vi "Periodic Tasks.vi"(8 "error in":errorcluster) -> ()   [LabVIEW 2016]
doc: "This VI runs in parallel to other tasks. It can contain as many user-defined periodic loops as you need. These can carry out PID or other sorts of timed response."
uses:
  <vilib>/Rock Robotics/WPI/DriverStation/WPI_DriverStationRobotMode2.ctl
  <vilib>/Rock Robotics/WPI/Utilities/WPI_GetSetVariantRefNum.vi
  <vilib>/Rock Robotics/Network Tables/NT Write Number.vi
  <vilib>/Instr/_visa.llb/VISA Configure Serial Port (Instr).vi
  Systems/Global 1.vi
  Global 2.vi
panel:
  in  "Gyro Reset":bool
  out "Angle":dbl
  in  "Reset Drive":bool
  out "Waveform Chart":dbl(graph)
  out "PSI":dbl=101.0986199
  out "Shoot 0":dbl format="%#_13g"
  out "Shoot 1":dbl format="%#_13g"
  out "read buffer":string="B:2,X:203.00"
  in  "Search_Params":string[](array[string])=["B", "X", "Y", "W1", "H1", "W2", "H2"]
  out "Last Complete Message":string="B:2,X:203.00,Y:125.00,W1:11,H1:27,W2:8,H2:25"
  out "length":i32=44
  in  "off set":dbl format="%#_13g"
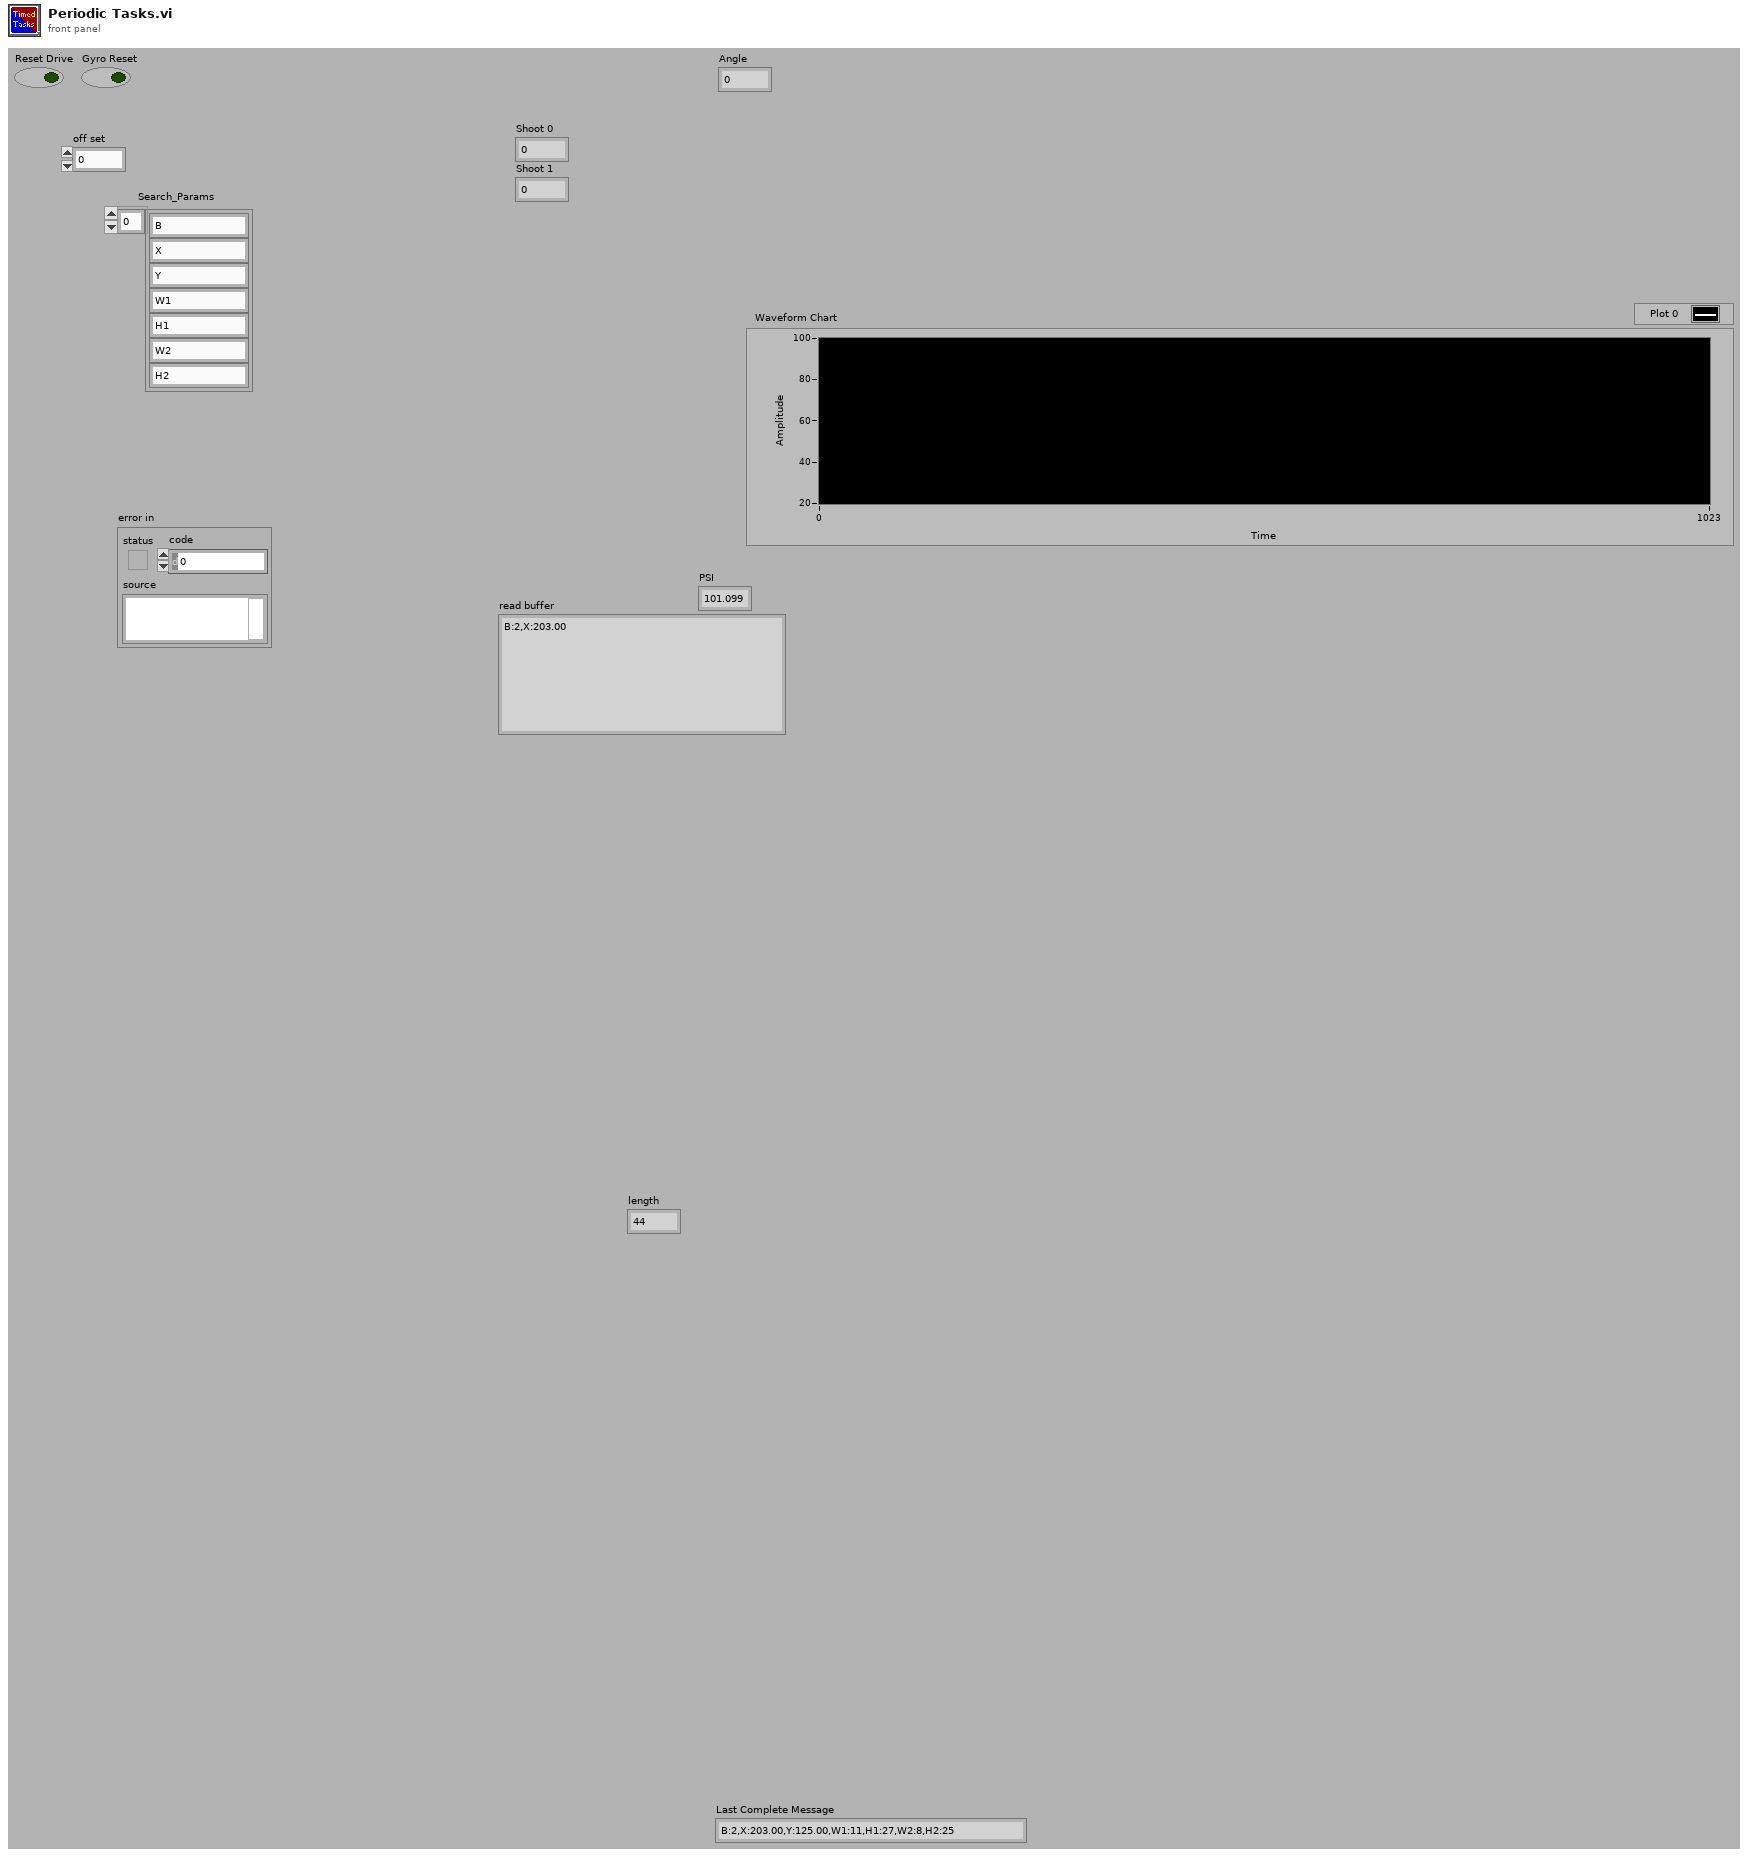
[diagram p1: front panel]
types:
  T1 = typedef "WPI_JoystickDevRef.ctl" = cluster{"Device":T2}
  T2 = typedef "WPI_JoystickDeviceEnum.ctl" = enum16{"USB 0", "USB 1", "USB 2", "USB 3", "USB 4", "USB 5"}
  T3 = typedef "WPI_MotorControlDeviceRef.ctl" = cluster{"DeviceStatus":errorcluster, "Type":T4, "PWM":cluster{"PWM Channel":T5, "DeadBand":T6}, "CAN":cluster{"Device Number":u8, "SetOutput VI Ref":variant, "GetOutput VI Ref":variant, "Enable VI Ref":variant, "Disable VI Ref":variant, "Data":variant}, "Invert":bool}
  T4 = typedef "WPI_MotorControlType.ctl" = enum16{"PWM", "CAN"}
  T5 = typedef "FPGA_DIOPWMChannel.ctl" = enum8{"PWM 0", "PWM 1", "PWM 2", "PWM 3", "PWM 4", "PWM 5", "PWM 6", "PWM 7", "PWM 8", "PWM 9", "PWM MXP 0", "PWM MXP 1", "PWM MXP 2", "PWM MXP 3", "PWM MXP 4", "PWM MXP 5", "PWM MXP 6", "PWM MXP 7", "PWM MXP 8", "PWM MXP 9", "Invalid"}
  T6 = typedef "WPI_PWMDeadband.ctl" = cluster{"Name":string, "maxPositivePwm":i32, "minPositivePwm":i32, "centerPwm":i32, "maxNegativePwm":i32, "minNegativePwm":i32, "angularRange":u16}
  T7 = typedef "WPI_CANTalonSRX_GlobalStatus.ctl" = cluster{"Applied Throttle":dbl, "Module Enabled":bool, "CAN Error":errorcluster, "Closed Loop Error":dbl, "Forward Limit Switch Closed":bool, "Reverse Limit Switch Closed":bool, "Sensor Position":dbl, "Sensor Velocity":dbl, "Current":dbl, "Sticky Fault - Over Temp":bool, "Sticky Fault - Under Voltage":bool, "Sticky Fault - Forward Limit":bool, "Sticky Fault - Reverse Limit":bool, "Sticky Fault - Forward Soft Limit":bool, "Sticky Fault - Reverse Soft Limit":bool, "Brake is Enabled":bool, "Encoder Position":dbl, "Encoder Velocity":dbl, "Encoder Index Count":dbl, "Encoder A Pin State":bool, "Encoder B Pin State":bool, "Encoder Index Pin State":bool, "Analog In":dbl, "Analog In Velocity":dbl, "Temperature (C)":dbl, "Battery Voltage":dbl, "Control 5 Is Supported":bool, "Current Profile Slot Select":dbl, "Pos Div 8":bool, "Vel Div 4":bool, "Pulse Width Position":i32, "Pulse Width Velocity":i32, "Pulse Width Rise To Rise (us)":i32, "Pulse Width Rise To Fall (us)":i32, "Mot Prof Active Is Under Run":bool, "Mot Prof Active Has Under Run":bool, "Mot Prof Active Is Last":bool, "Mot Prof Active Velocity Only":bool, "Mot Prof Active Is Valid":bool, "Mot Prof Buffer Is Full":bool, "Mot Prof Active Profile Slot Select":i32, "Mot Prof NextID":i32, "Mot Prof Count":i32, "Mot Prof Active Velocity":dbl, "Mot Prof Active Position":dbl, "Mot Prof Output Enable":i32}
  T8 = typedef "WPI_AnalogChannelDevRef.ctl" = cluster{"DevStatus":errorcluster, "Analog Channel":T9}
  T9 = typedef "FPGA_AIChannel.ctl" = enum8{"AI 0", "AI 1", "AI 2", "AI 3", "AI MXP 0", "AI MXP 1", "AI MXP 2", "AI MXP 3", "Invalid"}
  T10 = typedef "WPI_DriverStationRobotMode2.ctl" = enum16{"Autonomous Disabled", "Autonomous Enabled", "Teleop Disabled", "Teleop Enabled", "Disconnected", "Finish", "Test Disabled", "Test Enabled", "Emergency Stopped"}
  T11 = typedef "WPI_GyroDevRef.ctl" = cluster{"DevStatus":errorcluster, "Analog Channel":T9, "Offset":dbl, "Gain (VoltsPerDegree/Second)":dbl, "Gyro Type":enum16{"Analog", "XRS450"}, "Handle":i32, "SPI Bus":T12, "Device Found":bool, "Sample Rate":dbl, "Calibrate On Open":bool}
  T12 = typedef "spi_bus.ctl" = enum16{"SPI On-Board, CS0", "SPI On-Board, CS1", "SPI On-Board, CS2", "SPI On-Board, CS3", "SPI MXP", "Invalid"}
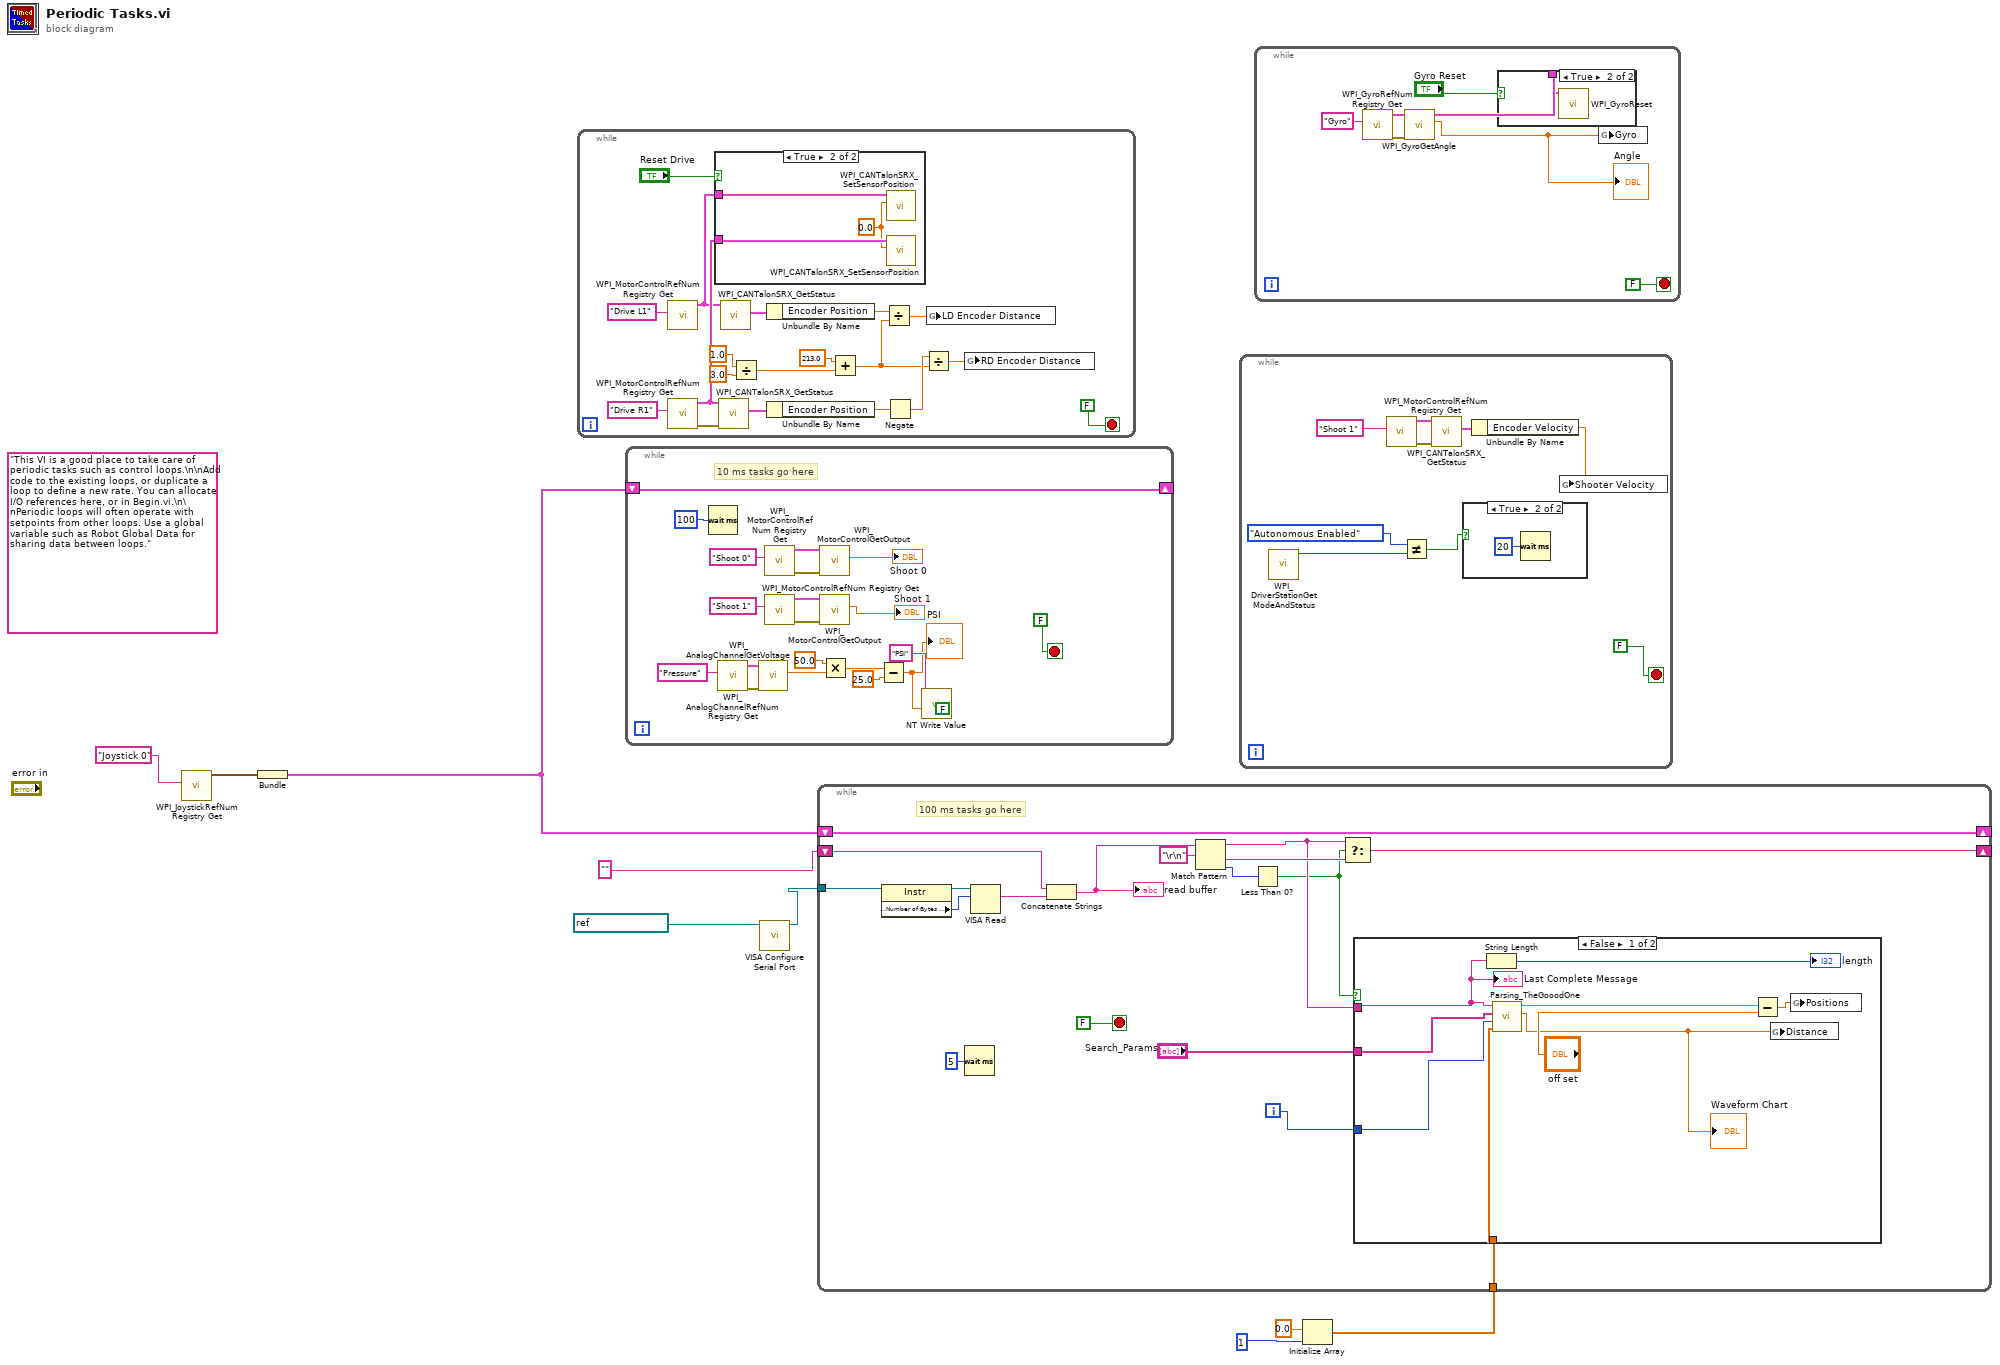
[diagram p0: block diagram]
diagram:
  (unwired) "This VI is a good place to take care of periodic tasks such as control loops.\n\nAdd code to the existing loops, or duplicate a loop to define a new rate. You can allocate I/O references here, or in Begin.vi.\n\nPeriodic loops will often operate with setpoints from other loops. Use a global variable such as Robot Global Data for sharing data between loops."
  n1 = call <vilib>:"WPI_JoystickRefNum Registry Get.vi"("refnum name"="Joystick 0") -> ("JoystickDevRef"=w2:T1)  [unwired: 1 in, 9 out]
  n2 = Bundle("JoystickDevRef"=w2) -> (w3:cluster{"JoystickDevRef":T1})  [unwired: 1 out]
  n3 = while {
    stop <- FALSE stop-if-true
    n4 = call <vilib>:"WPI_MotorControlRefNum Registry Get.vi"("refnum name"="Drive L1") -> ("MotorControlDevRef"=w21:T3)  [unwired: 9 in, 1 out]
    n5 = call <vilib>:"WPI_MotorControlRefNum Registry Get.vi"("refnum name"="Drive R1") -> ("error out"=w26:errorcluster, "MotorControlDevRef"=w22:T3)  [unwired: 9 in]
    n6 = case shown="True" "Reset Drive" {
      tunnel: w22 -> [_ w31]
      tunnel: w21 -> [_ w30]
      frame False {
      }
      frame True {
        w29 = 0.0
        n7 = call <vilib>:"WPI_CANTalonSRX_SetSensorPosition.vi"("New Sensor Position"=w29, "CAN Talon SRX Ref"=w30) -> ()  [unwired: 8 in, 2 out]
        n8 = call <vilib>:"WPI_CANTalonSRX_SetSensorPosition.vi"("New Sensor Position"=w29, "CAN Talon SRX Ref"=w31) -> ()  [unwired: 8 in, 2 out]
      }
    }
    n9 = call <vilib>:"WPI_CANTalonSRX_GetStatus.vi"("error in (no error)"=w26, "CAN Talon SRX Ref"=w22) -> ("Talon SRX Status"=w27:T7)  [unwired: 7 in, 2 out]
    n10 = call <vilib>:"WPI_CANTalonSRX_GetStatus.vi"("CAN Talon SRX Ref"=w21) -> ("Talon SRX Status"=w24:T7)  [unwired: 8 in, 2 out]
    n11 = Divide(x=1.0, y=3.0) -> (x/y=w16:dbl)
    n12 = Unbundle By Name(w24) -> ("Encoder Position"=w13:dbl)
    n13 = Unbundle By Name(w27) -> ("Encoder Position"=w19:dbl)
    n14 = Add(x=213.0, y=w16) -> (x+y=w12:dbl)
    n15 = Divide(x=w13, y=w12) -> (x/y=w11:dbl)
    n16 = Negate(x=w19) -> (-x=w14:dbl)
    n17 = Divide(x=w14, y=w12) -> (x/y=w10:dbl)
    n18 = global write "Global 2.vi" "LD Encoder Distance"(w11) -> ()
    n19 = global write "Global 2.vi" "RD Encoder Distance"(w10) -> ()
  }
  n20 = while {
    shift-right: [w49] -> _
    shift-left: w3 -> [w49]
    stop <- FALSE stop-if-true
    (unwired) FALSE
    # "10 ms tasks go here"
    n21 = Wait (ms)(milliseconds to wait=u32 100) -> ()  [unwired: 1 out]
    n22 = call <vilib>:"WPI_AnalogChannelRefNum Registry Get.vi"("refnum name"="Pressure") -> ("error out"=w40:errorcluster, "AIDeviceRef"=w39:T8)  [unwired: 9 in]
    n23 = call <vilib>:"WPI_AnalogChannelGetVoltage.vi"("error in (no error)"=w40, "AIDeviceRef"=w39) -> ("Voltage"=w37:dbl)  [unwired: 7 in, 2 out]
    n24 = call <vilib>:"WPI_MotorControlRefNum Registry Get.vi"("refnum name"="Shoot 0") -> ("error out"=w44:errorcluster, "MotorControlDevRef"=w48:T3)  [unwired: 9 in]
    n25 = call <vilib>:"WPI_MotorControlRefNum Registry Get.vi"("refnum name"="Shoot 1") -> ("error out"=w43:errorcluster, "MotorControlDevRef"=w45:T3)  [unwired: 9 in]
    n26 = call <vilib>:"WPI_MotorControlGetOutput.vi"("error in"=w44, "MotorControlDevRef"=w48) -> ("Output"=→"Shoot 0":dbl)  [unwired: 7 in, 2 out]
    n27 = call <vilib>:"WPI_MotorControlGetOutput.vi"("error in"=w43, "MotorControlDevRef"=w45) -> ("Output"=→"Shoot 1":dbl)  [unwired: 7 in, 2 out]
    n28 = Multiply(x=50.0, y=w37) -> (x*y=w35:dbl)
    n29 = Subtract(x=w35, y=25.0) -> (x-y=w32:dbl)
    "PSI" <- w32
    n30 = call-poly <vilib>:"NT Write Value.vi"("Numeric"=w32, "Name"="PSI") -> ()  [unwired: 9 in, 1 out]
  }
  n31 = call-poly "VISA Configure Serial Port"("VISA resource name"=refnum<visa-resource-name> "ASRL2::INSTR") -> ("VISA resource name out"=w5:refnum<visa-resource-name>)  [unwired: 13 in, 1 out]
  n32 = while {
    stop <- FALSE stop-if-true
    n33 = call <vilib>:"WPI_DriverStationGetModeAndStatus.vi"() -> ("Robot Mode"=w54:T10)  [unwired: 10 in, 1 out]
    n34 = call <vilib>:"WPI_MotorControlRefNum Registry Get.vi"("refnum name"="Shoot 1") -> ("error out"=w58:errorcluster, "MotorControlDevRef"=w59:T3)  [unwired: 9 in]
    n35 = Not Equal?(x=WPI_DriverStationRobotMode2."Autonomous Enabled" ("Robot Mode"), y=w54) -> (x != y?=w52:bool)
    n36 = call <vilib>:"WPI_CANTalonSRX_GetStatus.vi"("error in (no error)"=w58, "CAN Talon SRX Ref"=w59) -> ("Talon SRX Status"=w57:T7)  [unwired: 7 in, 2 out]
    n37 = case shown="True" w52 {
      frame False {
      }
      frame True {
        n38 = Wait (ms)(milliseconds to wait=u32 20) -> ()  [unwired: 1 out]
      }
    }
    n39 = Unbundle By Name(w57) -> ("Encoder Velocity"=w56:dbl)
    n40 = global write "Global 2.vi" "Shooter Velocity"(w56) -> ()
  }
  n41 = while {
    stop <- FALSE stop-if-true
    n42 = call <vilib>:"WPI_GyroRefNum Registry Get.vi"("refnum name"="Gyro") -> ("error out"=w65:errorcluster, "GyroDevRef"=w68:T11)  [unwired: 9 in]
    n43 = call <vilib>:"WPI_GyroGetAngle.vi"("error in"=w65, "GyroDevRef"=w68) -> ("Angle"=w62:dbl, "GyroDevRef"=w64:T11)  [unwired: 5 in, 3 out]
    "Angle" <- w62
    n44 = case shown="True" "Gyro Reset" {
      tunnel: w64 -> [_ w69]
      frame False {
      }
      frame True {
        n45 = call <vilib>:"WPI_GyroReset.vi"("GyroDevRef"=w69) -> ()  [unwired: 9 in, 2 out]
      }
    }
    n46 = global write "Global 2.vi" "Gyro"(w62) -> ()
  }
  n47 = Initialize Array(0.0 ("element"), 1) -> (w9:dbl[])
  n48 = while {
    shift-right: [w86] -> _
    shift-left: w3 -> [w86]
    tunnel: w5 -> [w81]
    shift-right: [w73] -> _
    shift-left: "" -> [w80]
    tunnel: w9 -> [w70]
    i -> [w71]
    stop <- FALSE stop-if-true
    # "100 ms tasks go here"
    n49 = property class="Instr"(reference=w81) -> (reference out=w85:refnum<visa-resource-name>, "Serial Settings:Number of Bytes at Serial Port"=w84:u32)  [unwired: 1 in, 1 out]
    n50 = Wait (ms)(milliseconds to wait=u32 5) -> ()  [unwired: 1 out]
    n51 = VISA Read(VISA resource name=w85, byte count=w84) -> (read buffer=w79:string)  [unwired: 1 in, 3 out]
    n52 = Concatenate Strings(w80, w79) -> (w78:string)
    "read buffer" <- w78
    n53 = Match Pattern(string=w78, regular expression="\r\n") -> (before substring=w74:string, after substring=w75:string, offset past match=w76:i32)  [unwired: 1 in, 1 out]
    n54 = Less Than 0?(x=w76) -> (x < 0?=w72:bool)
    n55 = Select(t=w74, s=w72, f=w75) -> (s? t:f=w73:string)
    n56 = case shown="False" w72 {
      tunnel: "Search_Params" -> [w95 _]
      tunnel: w74 -> [w94 _]
      tunnel: w71 -> [w90 _]
      tunnel: w70 -> [w89 _]
      frame False {
        n57 = String Length(string=w94) -> (length=→"length":i32)
        n58 = call "Parsing_TheGooodOne.vi"("array"=w89, "Iterations"=w90, "Search_Params"=w95, "Input"=w94) -> ("Corrected distance"=w88:dbl, "Value-Reference"=w93:dbl)  [unwired: 4 in]
        "Waveform Chart" <- w88
        n59 = Subtract(x=w93, y="off set") -> (x-y=w91:dbl)
        n60 = global write "Global 1.vi" "Distance"(w88) -> ()
        n61 = global write "Global 1.vi" "Positions"(w91) -> ()
        "Last Complete Message" <- w94
      }
      frame True {
      }
    }
  }
